vi "Change Channel Name.vi"(9 "Channel Units":T1, 10 "Channel Names":T2, 11 "readable in":refnum<class "Readable.lvclass">) -> (3 "readable out":refnum<class "Readable.lvclass">)   [LabVIEW 2017, in "Readable.lvclass"]
uses:
  Readable.lvclass
  Channel Names.ctl
  Channel Units.ctl
  Readable.lvclass/Readable.ctl
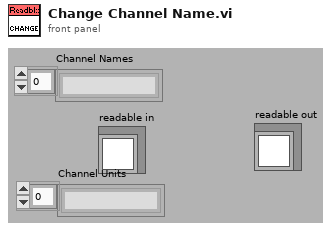
[diagram p1: front panel]
types:
  T1 = typedef "Readable.lvclass/Channel Units.ctl" = string[]
  T2 = typedef "Readable.lvclass/Channel Names.ctl" = string[]
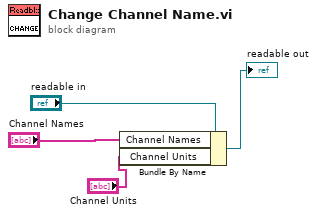
[diagram p0: block diagram]
diagram:
  n1 = Bundle By Name(cluster="readable in", "Channel Names"="Channel Names", "Channel Units"="Channel Units") -> (→"readable out":refnum<class "Readable.lvclass">)
